vi "newTarget2.vi"(8 "error in (no error)":errorcluster, 9 "Target Y":dbl, 10 "Target X":dbl) -> (0 "error out":errorcluster, 1 "Target y":dbl, 2 "Target x":dbl, 3 "NewTarget":bool)   [LabVIEW 2017, in "admittanceControllerLibrary.lvlib"]
doc: "This VI etsablishes whether the target is new. A boolean is output in the case of a new target so that the PID Integral can be reset to prevent PID windup."
uses:
  admittanceControllerLibrary.lvlib
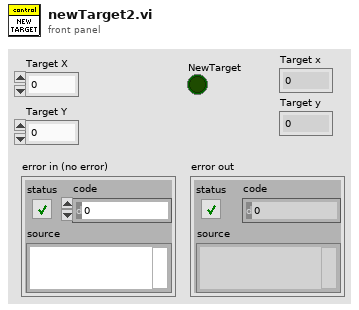
[diagram p1: front panel]
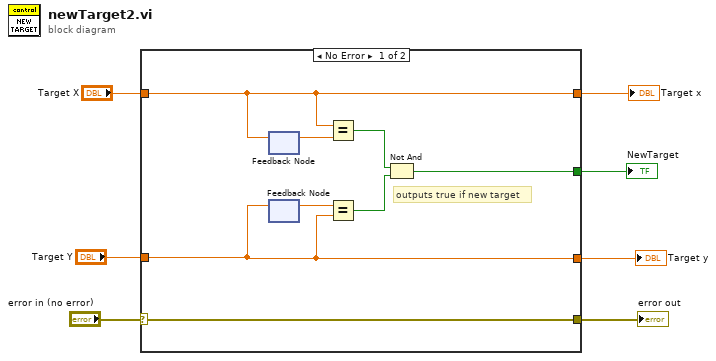
[diagram p0: block diagram]
diagram:
  n1 = case shown="No Error" "error in (no error)" {
    selector: "error in (no error)" -> [w9 w17]
    tunnel: "Target X" -> [w11 w18]
    tunnel: "Target Y" -> [w10 w16]
    tunnel: [w11 w18] -> w5
    tunnel: [w10 w16] -> w4
    tunnel: [w9 w17] -> w2
    tunnel: [w8 _] -> w1
    frame No Error {
      # "outputs true if new target"
      n2 = feedback #1() -> (w13:dbl)  [unwired: 1 in]
      n3 = feedback-in #1(w11) -> ()
      n4 = feedback #2() -> (w12:dbl)  [unwired: 1 in]
      n5 = feedback-in #2(w10) -> ()
      n6 = Equal?(x=w11, y=w13) -> (x = y?=w15:bool)
      n7 = Equal?(x=w12, y=w10) -> (x = y?=w14:bool)
      n8 = Not And(1:w14, 2:w15) -> (0:w8:bool)
    }
    frame Error {
    }
  }
  "error out" <- w2
  "Target x" <- w5
  "Target y" <- w4
  "NewTarget" <- w1
